vi "New CHM Wizard.vi"(7 "Project:Active Project":refnum<vi>, 9 "Title":string, 11 "Base CHM Directory":path) -> ()   [LabVIEW 2015]
uses:
  Wizard State.ctl
  <vilib>/Utility/config.llb/Write Key (String).vi
  <vilib>/Utility/config.llb/Write Key (Path).vi
  <vilib>/Utility/config.llb/NI_LVConfig.lvlib
panel:
  in  "Tab Control":T1(tab)
  in  "Default Topic Name":string
  in  "Additional Pages":string[](array[string])
  out "error out":errorcluster
  in  "Previous":bool
  in  "Cancel":bool
  in  "Next":bool
  # "Welcome to the Compiled Help Menu Wizard."
  # "This will add the CHM Generator to your project and create a new auto-populating folder\nfor your Compiled Help Menu source files."
  # "Choose a title for your Compiled Help Menu"
  # "Choose an empty directory for your Compiled  HTML Help source files."
  # "Choose a name for the default topic of your Compiled HTML Help file. \nThis will be generated in the directory you specified."
  # "List any other pages you would like to generate on creation. You can add\nother pages later by placing them in the source directory."
  # "A critical error occured!"
  # "#TODO fill in contact info, report error?"
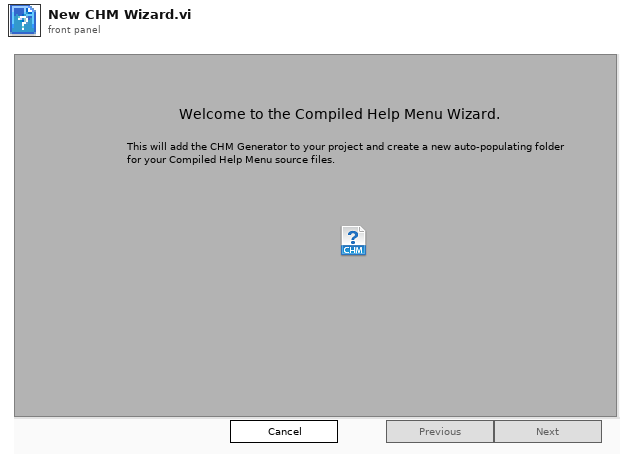
[diagram p1: front panel]
types:
  T1 = enum32{"Welcome", "Choose CHM Title", "Choose Base Path", "Choose Default Topic Name", "Other Pages", "Done", "Error"}
  T2 = typedef "Wizard State.ctl" = enum16{"Initialize", "Wait for User", "Finish"}
  T3 = enum32{"Invalid", "Standard", "Closed", "Hidden", "Minimized", "Maximized"}
  T4 = enum32{"Welcome", "Choose CHM Title", "Choose Base Path", "Choose Default Topic Name"}
  T5 = enum8{"Enabled", "Disabled", "Disabled and Grayed Out"}
  T6 = typedef "NI_LVConfig.lvlib/Config Data RefNum.ctl" = refnum<k1>
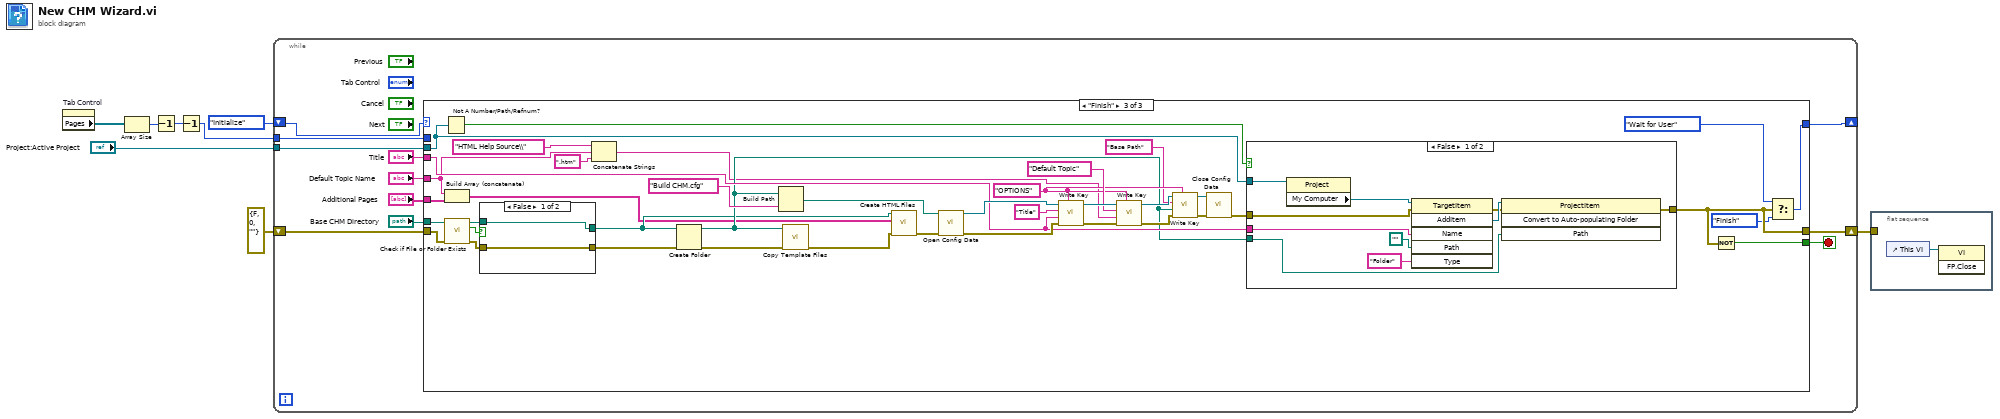
[diagram p0: block diagram]
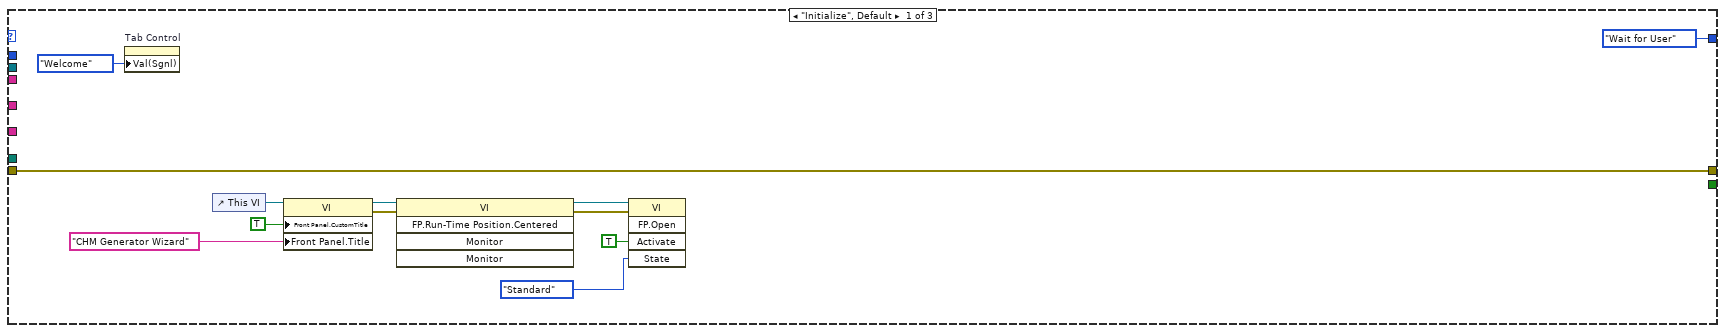
[diagram p2: hidden frame]
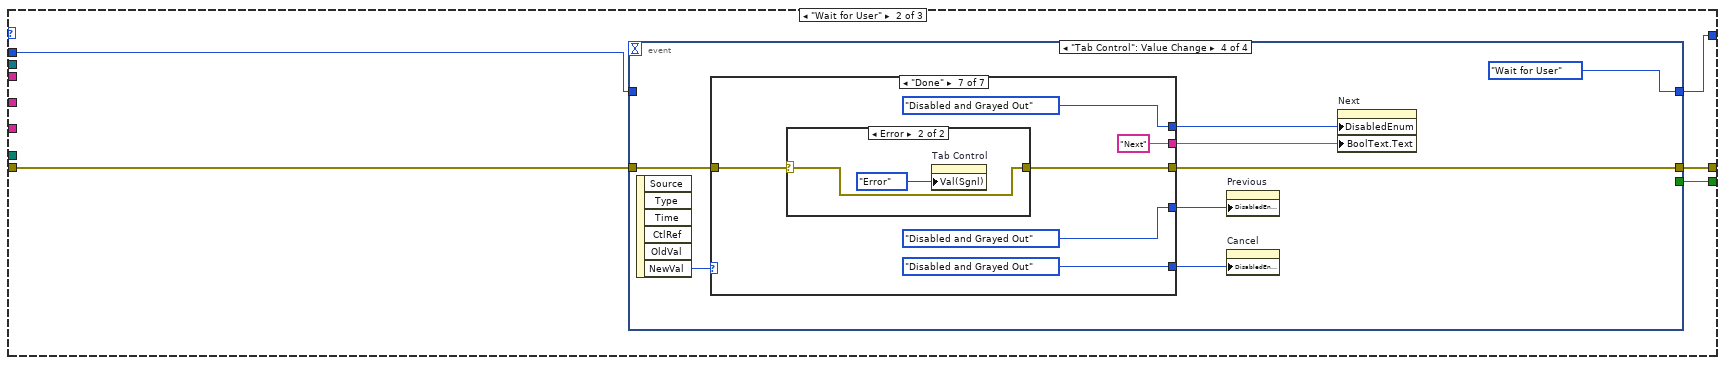
[diagram p3: hidden frame]
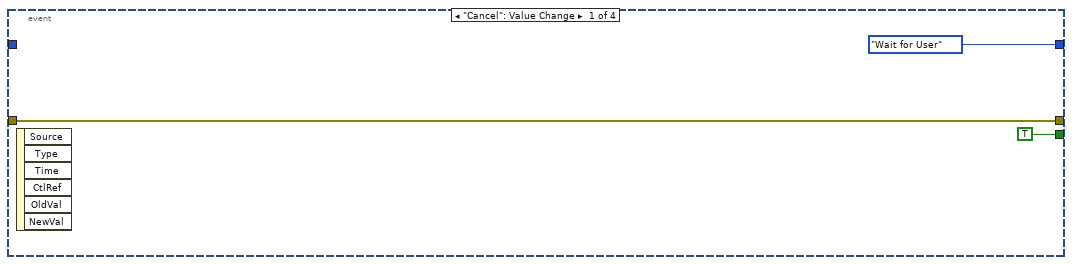
[diagram p4: hidden frame]
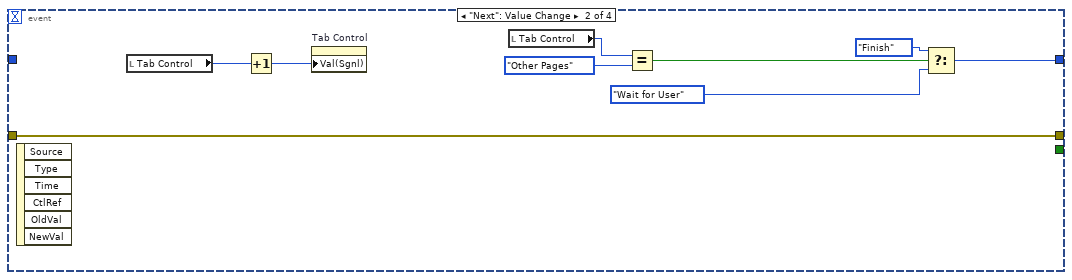
[diagram p5: hidden frame]
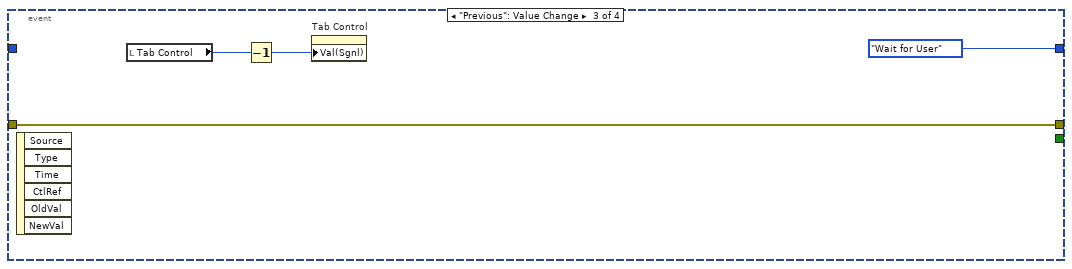
[diagram p6: hidden frame]
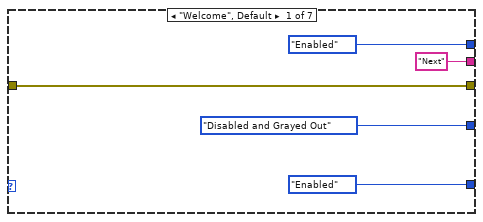
[diagram p7: hidden frame]
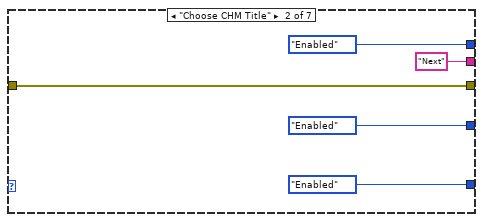
[diagram p8: hidden frame]
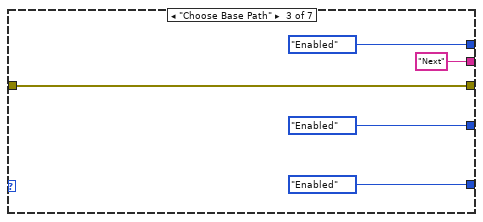
[diagram p9: hidden frame]
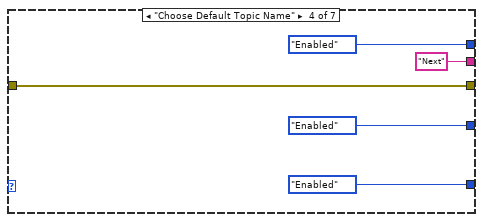
[diagram p10: hidden frame]
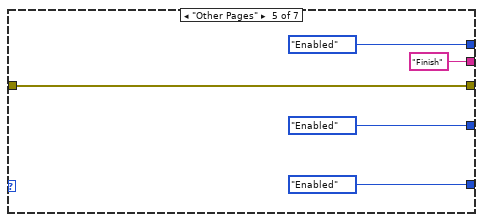
[diagram p11: hidden frame]
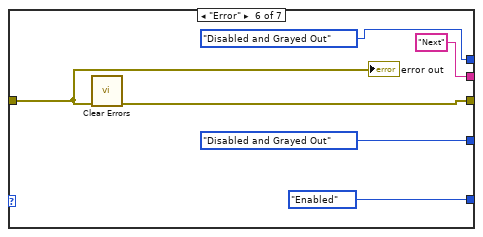
[diagram p12: hidden frame]
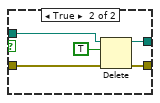
[diagram p15: hidden frame]
diagram:
  n1 = property on="Tab Control" class="TabCtl (strict)"() -> ("Pages"=w7:refnum<vi>[])  [unwired: 2 in, 2 out]
  n2 = Array Size(array=w7) -> (size(s)=w6:i32)
  n3 = Decrement(x=w6) -> (x-1=w3:i32)
  n4 = Decrement(x=w3) -> (x-1=w2:i32)
  n5 = while {
    shift-right: [w18] -> _
    shift-left: Wizard_State."Initialize" -> [w19]
    tunnel: w2 -> [w16]
    shift-right: [w12] -> w1
    shift-left: errorcluster {"status"=FALSE, "code"=0, "source"=""} ("error out") -> [w11]
    tunnel: "Project:Active Project" -> [w10]
    stop <- w17 stop-if-true
    n6 = case shown="\"Finish\"" w19 {
      tunnel: [Wizard_State."Wait for User" w35 w105] -> w18
      tunnel: [_ w36 w111] -> w17
      tunnel: w16 -> [_ w34 _]
      tunnel: "Base CHM Directory" -> [_ _ w140]
      tunnel: "Title" -> [_ _ w121]
      tunnel: "Default Topic Name" -> [_ _ w104]
      tunnel: [w21 w33 w108] -> w12
      tunnel: w11 -> [w21 w32 w122]
      tunnel: w10 -> [_ _ w119]
      tunnel: "Additional Pages" -> [_ _ w110]
      frame "Initialize", Default {
        n7 = property on="Tab Control" class="TabCtl (strict)"("Val(Sgnl)"=T4."Welcome" ("Tab Control")) -> ()  [unwired: 2 in, 2 out]
        n8 = control-ref of="This VI"() -> (w29:refnum<vi>)
        n9 = property class="VI"(reference=w29, "Front Panel.CustomTitle"=TRUE ("Front Panel Window:Custom Title"), "Front Panel.Title"="CHM Generator Wizard" ("Front Panel Window:Title")) -> (reference out=w27:refnum<vi>, error out=w26:errorcluster)  [unwired: 1 in]
        n10 = invoke class="VI" method="FP.Run-Time Position.Centered"(reference=w27, error in=w26) -> (reference out=w25:refnum<vi>, error out=w24:errorcluster)  [unwired: 3 in, 3 out]
        n11 = invoke class="VI" method="FP.Open"(reference=w25, error in=w24, "Activate"=TRUE ("Activate?"), "State"=T3."Standard") -> ()  [unwired: 1 in, 5 out]
      }
      frame "Wait for User" {
        n12 = event shown="[3] \"Tab Control\": Value Change" {
          selector: _ -> [_ _ _ _]
          dyn-events: _ -> [_ _ _ _]
          timeout: _ -> [_ _ _ _]
          tunnel: [TRUE _ _ _] -> w36
          tunnel: [Wizard_State."Wait for User" w42 Wizard_State."Wait for User" Wizard_State."Wait for User"] -> w35
          tunnel: w34 -> [_ _ _ _]
          tunnel: w32 -> [w37 w41 w49 w57]
          tunnel: [w37 w41 w49 w56] -> w33
          event "Cancel": Value Change {
            n13 = event-data() -> ()  [unwired: 1 in, 6 out]
          }
          event "Next": Value Change {
            n14 = event-data() -> ()  [unwired: 1 in, 6 out]
            n15 = local read "Tab Control"() -> (w48:T1)
            n16 = Increment(x=w48) -> (x+1=w47:T1)
            n17 = property on="Tab Control" class="TabCtl (strict)"("Val(Sgnl)"=w47) -> ()  [unwired: 2 in, 2 out]
            n18 = local read "Tab Control"() -> (w46:T1)
            n19 = Equal?(x=w46, y=T1."Other Pages") -> (x = y?=w43:bool)
            n20 = Select(t=Wizard_State."Finish", s=w43, f=Wizard_State."Wait for User") -> (s? t:f=w42:T2)
          }
          event "Previous": Value Change {
            n21 = event-data() -> ()  [unwired: 1 in, 6 out]
            n22 = local read "Tab Control"() -> (w52:T1)
            n23 = Decrement(x=w52) -> (x-1=w51:T1)
            n24 = property on="Tab Control" class="TabCtl (strict)"("Val(Sgnl)"=w51) -> ()  [unwired: 2 in, 2 out]
          }
          event "Tab Control": Value Change {
            n25 = event-data() -> ("NewVal"=w59:T1)  [unwired: 1 in, 5 out]
            n26 = case shown="\"Done\"" w59 {
              tunnel: [T5."Disabled and Grayed Out" ("t") T5."Enabled" ("t") T5."Enabled" ("t") T5."Enabled" ("t") T5."Enabled" ("t") T5."Disabled and Grayed Out" ("t") T5."Disabled and Grayed Out" ("t")] -> w58
              tunnel: ["Next" "Next" "Next" "Next" "Finish" "Next" "Next"] -> w53
              tunnel: w57 -> [w63 w68 w73 w78 w83 w89 w93]
              tunnel: [w63 w68 w73 w78 w83 w88 w92] -> w56
              tunnel: [T5."Enabled" ("t") T5."Enabled" ("t") T5."Enabled" ("t") T5."Enabled" ("t") T5."Enabled" ("t") T5."Disabled and Grayed Out" ("t") T5."Disabled and Grayed Out" ("t")] -> w55
              tunnel: [T5."Enabled" ("t") T5."Enabled" ("t") T5."Enabled" ("t") T5."Enabled" ("t") T5."Enabled" ("t") T5."Enabled" ("t") T5."Disabled and Grayed Out" ("t")] -> w54
              frame "Welcome", Default {
              }
              frame "Choose CHM Title" {
              }
              frame "Choose Base Path" {
              }
              frame "Choose Default Topic Name" {
              }
              frame "Other Pages" {
              }
              frame "Error" {
                n27 = call <vilib>:"Clear Errors.vi"("error in (no error)"=w89) -> ("error out"=w88:errorcluster)  [unwired: 5 in, 1 out]
                "error out" <- w89
              }
              frame "Done" {
                n28 = case shown="Error" w93 {
                  selector: w93 -> [w98 w99]
                  tunnel: [w98 w99] -> w92
                  frame No Error {
                  }
                  frame Error {
                    n29 = property on="Tab Control" class="TabCtl (strict)"("Val(Sgnl)"=T1."Error" ("Value (Signaling)")) -> ()  [unwired: 2 in, 2 out]
                  }
                }
              }
            }
            n30 = property on="Previous" class="Bool"("DisabledEnum"=w58) -> ()  [unwired: 2 in, 2 out]
            n31 = property on="Cancel" class="Bool"("DisabledEnum"=w54) -> ()  [unwired: 2 in, 2 out]
            n32 = property on="Next" class="Bool"("DisabledEnum"=w55, "BoolText.Text"=w53) -> ()  [unwired: 2 in, 2 out]
          }
        }
      }
      frame "Finish" {
        w131 = "OPTIONS" ("section")
        n33 = Not A Number/Path/Refnum?(number/path/refnum=w119) -> (NaN/Path/Refnum?=w118:bool)
        n34 = Build Array (concatenate)(w104, w110) -> (w109:string[])
        n35 = call <vilib>:"Check if File or Folder Exists.vi"("error in (no error)"=w122, "path"=w140) -> ("error out"=w123:errorcluster, "file or folder exists?"=w138:bool, "dup path"=w139:path)  [unwired: 7 in]
        n36 = case shown="False" w138 {
          tunnel: w139 -> [w153 w157]
          tunnel: [w153 w156] -> w114
          tunnel: [w152 w155] -> w124
          tunnel: w123 -> [w152 w154]
          frame False {
          }
          frame True {
            n37 = Delete(path (use dialog)=w157, entire hierarchy (F)=TRUE, error in=w154) -> (deleted path=w156:path, error out=w155:errorcluster)  [unwired: 2 in, 1 out]
          }
        }
        n38 = Concatenate Strings("HTML Help Source\\" ("string"), w104, ".htm" ("string")) -> (w102:string)
        n39 = Create Folder(path (use dialog)=w114, error in=w124) -> (created path=w116:path, error out=w125:errorcluster)  [unwired: 1 in, 1 out]
        n40 = Build Path(base path=w116, name or relative path="Build CHM.cfg") -> (appended path=w115:path)
        n41 = call "Copy Template Files.vi"("error in (no error)"=w125, "Base Path"=w116) -> ("error out"=w113:errorcluster)  [unwired: 9 in]
        n42 = call "Create HTML Files.vi"("error in (no error)"=w113, "Topics"=w109, "path"=w114) -> ("error out"=w112:errorcluster)  [unwired: 8 in]
        n43 = call <vilib>:"Open Config Data.vi"("error in (no error)"=w112, "configuration file path"=w115) -> ("error out"=w137:errorcluster, "refnum"=w136:T6)  [unwired: 7 in, 1 out]
        n44 = call-poly <vilib>:"Write Key.vi"("section"=w131, "error in (no error)"=w137, "value"=w121, "key"="Title", "refnum"=w136) -> ("error out"=w134:errorcluster, "refnum out"=w133:T6)  [unwired: 4 in, 1 out]
        n45 = call-poly <vilib>:"Write Key.vi"("section"=w131, "error in (no error)"=w134, "value"=w102, "key"="Default Topic", "refnum"=w133) -> ("error out"=w130:errorcluster, "refnum out"=w128:T6)  [unwired: 4 in, 1 out]
        n46 = call-poly <vilib>:"Write Key.vi"("section"=w131, "error in (no error)"=w130, "value"=w116, "key"="Base Path", "refnum"=w128) -> ("error out"=w129:errorcluster, "refnum out"=w127:T6)  [unwired: 4 in, 1 out]
        n47 = call <vilib>:"Close Config Data.vi"("error in (no error)"=w129, "refnum"=w127) -> ("error out"=w120:errorcluster)  [unwired: 8 in, 1 out]
        n48 = case shown="False" w118 {
          tunnel: w121 -> [w148 _]
          tunnel: w116 -> [w144 _]
          tunnel: w120 -> [w147 w151]
          tunnel: [w142 w151] -> w108
          tunnel: w119 -> [w146 _]
          frame False {
            n49 = property class="Project"(reference=w146) -> ("My Computer"=w150:refnum<vi>)  [unwired: 1 in, 2 out]
            n50 = invoke class="TargetItem" method="AddItem"(reference=w150, error in=w147, "Name"=w148, "Path"=path "", "Type"="Folder") -> (error out=w143:errorcluster, "AddItem"=w145:refnum<vi>)  [unwired: 1 in, 4 out]
            n51 = invoke class="ProjectItem" method="Convert to Auto-populating Folder"(reference=w145, error in=w143, "Path"=w144) -> (error out=w142:errorcluster)  [unwired: 1 in, 3 out]
          }
          frame True {
          }
        }
        n52 = Not(x=w108) -> (.not. x?=w111:bool)
        n53 = Select(t=Wizard_State."Wait for User", s=w108, f=Wizard_State."Finish") -> (s? t:f=w105:T2)
      }
    }
  }
  n54 = flat-sequence {
    tunnel: w1 -> [_]
    frame #0 {
      n55 = control-ref of="This VI"() -> (w159:refnum<vi>)
      n56 = invoke class="VI" method="FP.Close"(reference=w159) -> ()  [unwired: 2 in, 3 out]
    }
  }
